vi "Filtre items.vi"(6 "filtre":string, 8 "item list":string[](array[string])) -> (0 "# match":i32, 2 "filtred list":string[](array[string]))   [LabVIEW 2010, in "magic ring.xctl"]
uses:
  magic ring.xctl
  controls/filtre type.ctl
  <vilib>/regexp/Match Regular Expression.xnode
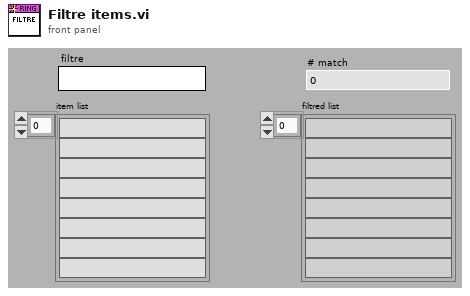
[diagram p1: front panel]
types:
  T1 = typedef "filtre type.ctl" = enum16{"no star", "start with star", "contain star"}
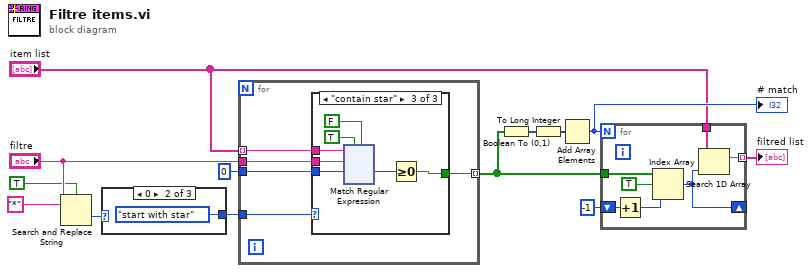
[diagram p0: block diagram]
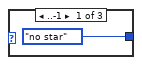
[diagram p2: hidden frame]
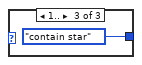
[diagram p3: hidden frame]
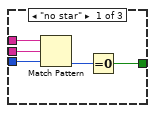
[diagram p4: hidden frame]
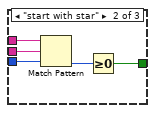
[diagram p5: hidden frame]
diagram:
  n1 = Search and Replace String(case sensitive?=TRUE, input string="filtre", search string="*") -> (offset past replacement=w11:i32)  [unwired: 5 in, 3 out]
  n2 = case shown="0" w11 {
    tunnel: [filtre_type."no star" filtre_type."start with star" filtre_type."contain star"] -> w10
    frame ..-1 {
    }
    frame 0 {
    }
    frame 1.. {
    }
  }
  n3 = for {
    tunnel: "item list" -> [w21] mode=indexing
    tunnel: "filtre" -> [w20]
    tunnel: w10 -> [w17]
    tunnel: [w18] -> w5 mode=indexing
    tunnel: 0 -> [w19]
    n4 = case shown="\"contain star\"" w17 {
      tunnel: w21 -> [w26 w31 w35]
      tunnel: w20 -> [w25 w30 w38]
      tunnel: w19 -> [w24 w29 w37]
      tunnel: [w22 w27 w36] -> w18
      frame "no star" {
        n5 = Match Pattern(string=w26, regular expression=w25, offset (0)=w24) -> (offset past match=w23:i32)  [unwired: 3 out]
        n6 = Equal To 0?(x=w23) -> (x = 0?=w22:bool)
      }
      frame "start with star" {
        n7 = Match Pattern(string=w31, regular expression=w30, offset (0)=w29) -> (offset past match=w28:i32)  [unwired: 3 out]
        n8 = Greater Or Equal To 0?(x=w28) -> (x >= 0?=w27:bool)
      }
      frame "contain star" {
        n9 = xnode "Match Regular Expression"("input string"=w35, "regular expression"=w38, "offset (0)"=w37, "ignore case? (F)"=TRUE, "multiline? (F)"=FALSE) -> ("offset past match"=w34:i32)  [unwired: 1 in, 4 out]
        n10 = Greater Or Equal To 0?(x=w34) -> (x >= 0?=w36:bool)
      }
    }
  }
  n11 = Boolean To (0,1)(Boolean=w5) -> (0, 1=w8:i16[])
  n12 = To Long Integer(number=w8) -> (32bit integer=w9:i32[])
  n13 = Add Array Elements(numeric array=w9) -> (sum=w7:i32)
  "# match" <- w7
  n14 = for {
    N: w7 -> [_]
    tunnel: "item list" -> [w152]
    tunnel: w5 -> [w156]
    shift-right: [w153] -> _
    shift-left: -1 ("start index (0)") -> [w154]
    tunnel: [w151] -> w4 mode=indexing
    n15 = Increment(x=w154) -> (x+1=w150:i32)
    n16 = Search 1D Array(1D array=w156, element=TRUE, start index (0)=w150) -> (index of element=w153:i32)
    n17 = Index Array(array=w152, index=w153) -> (element=w151:string)
  }
  "filtred list" <- w4
